vi "Inicio.vi"() -> ()   [LabVIEW 2025]
panel:
  in  "stop":bool
  in  "OK Button":bool
  # "Bienvenido a Smartchef"
  # "Su sistema automatizado y su interfaz intuitiva te permiten \nmezclar, batir y crear como un verdadero chef, \nsin complicaciones."
  # "Haz clic en “Iniciar” y descubre cómo SmartChef transforma \nla forma en que cocinas."
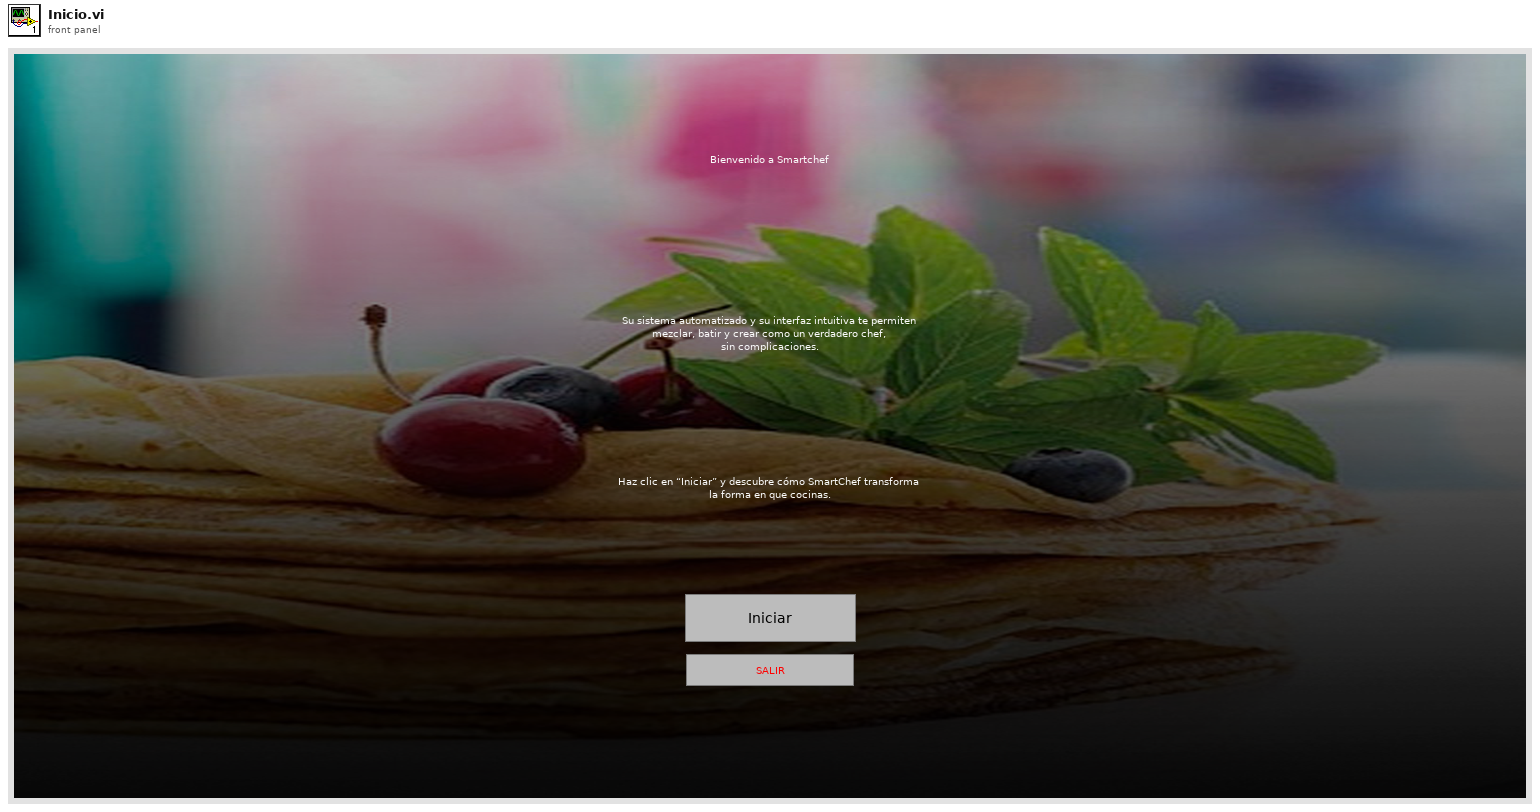
[diagram p1: front panel]
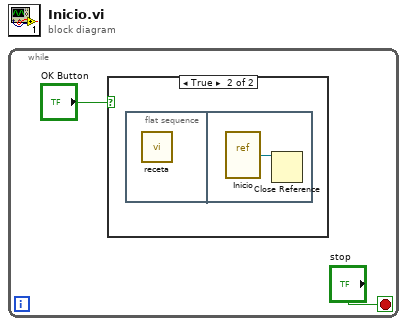
[diagram p0: block diagram]
diagram:
  n1 = while {
    stop <- "stop" stop-if-true
    n2 = case shown="True" "OK Button" {
      frame False {
      }
      frame True {
        n3 = flat-sequence {
          frame #0 {
            n4 = call "receta.vi"() -> ()  [unwired: 12 in]
          }
          frame #1 {
            n5 = vi-ref "Inicio.vi"() -> (w3:refnum<vi>)
            n6 = Close Reference(reference=w3) -> ()  [unwired: 1 in, 1 out]
          }
        }
      }
    }
  }
